vi "Do Draw.vi"(9 "color":u32(colorbox), 10 "picture in":picture, 11 "Square Message":refnum<class "Square Message.lvclass">) -> (2 "picture out":picture)   [LabVIEW 2019, in "Draw Messages.lvlib" / "Square Message.lvclass"]
doc: "Draw whatever the message needs to draw into the picture."
uses:
  Square Message.lvclass
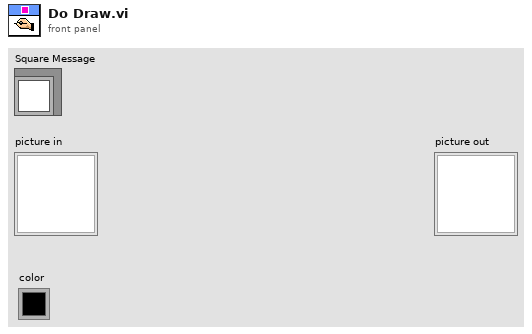
[diagram p1: front panel]
types:
  T1 = cluster{"left":i16, "top":i16, "right":i16, "bottom":i16}
  T2 = cluster{"number: 0 to 1":dbl, "number: 0 to 1":dbl}
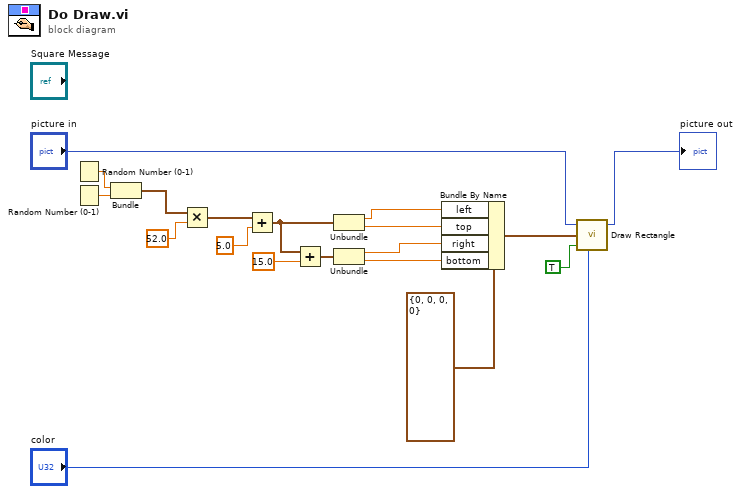
[diagram p0: block diagram]
diagram:
  n1 = Random Number (0-1)() -> (number: 0 to 1=w18:dbl)
  n2 = Random Number (0-1)() -> (number: 0 to 1=w17:dbl)
  n3 = Bundle("number: 0 to 1"=w18, "number: 0 to 1"=w17) -> (w16:T2)  [unwired: 1 in]
  n4 = Multiply(x=w16, y=52.0) -> (x*y=w15:T2)
  n5 = Add(x=w15, y=5.0) -> (x+y=w9:T2)
  n6 = Add(x=w9, y=15.0) -> (x+y=w7:T2)
  n7 = Unbundle(w9) -> ("number: 0 to 1"=w5:dbl, "number: 0 to 1"=w4:dbl)
  n8 = Unbundle(w7) -> ("number: 0 to 1"=w3:dbl, "number: 0 to 1"=w2:dbl)
  n9 = Bundle By Name(cluster=T1 {"left"=0, "top"=0, "right"=0, "bottom"=0} ("rect"), "left"=w5, "top"=w4, "right"=w3, "bottom"=w2) -> (w1:T1)
  n10 = call <vilib>:"Draw Rectangle.vi"("picture"="picture in", "rect"=w1, "fill?(F)"=TRUE, "color(black)"="color") -> ("new picture"=→"picture out":picture)  [unwired: 5 in]
